vi "1dparse.vi"(5 "max0 2":u16, 7 "min0 2":u16, 10 "channel number":T1, 11 "2d intensity array output 2":i32[][](array[numeric])) -> (3 "2d intensity array output":i32[][](array[numeric]))   [LabVIEW 2016]
uses:
  controls/1d gate selection.ctl
  Drivers/Pixie4DLL.dll
panel:
  out "size(s)":i32
  out "data0":u16[](array[numeric])
  out "timeb3":u16[](array[numeric])
  out "timeb2":u16[](array[numeric])
  out "timeb1":u16[](array[numeric])
  out "timeb0":u16[](array[numeric])
  out "datab3":u16[](array[numeric])
  out "datab2":u16[](array[numeric])
  out "datab1":u16[](array[numeric])
  out "return type":u32
  out "subarray":i32[](array[numeric])
  out "size":u16
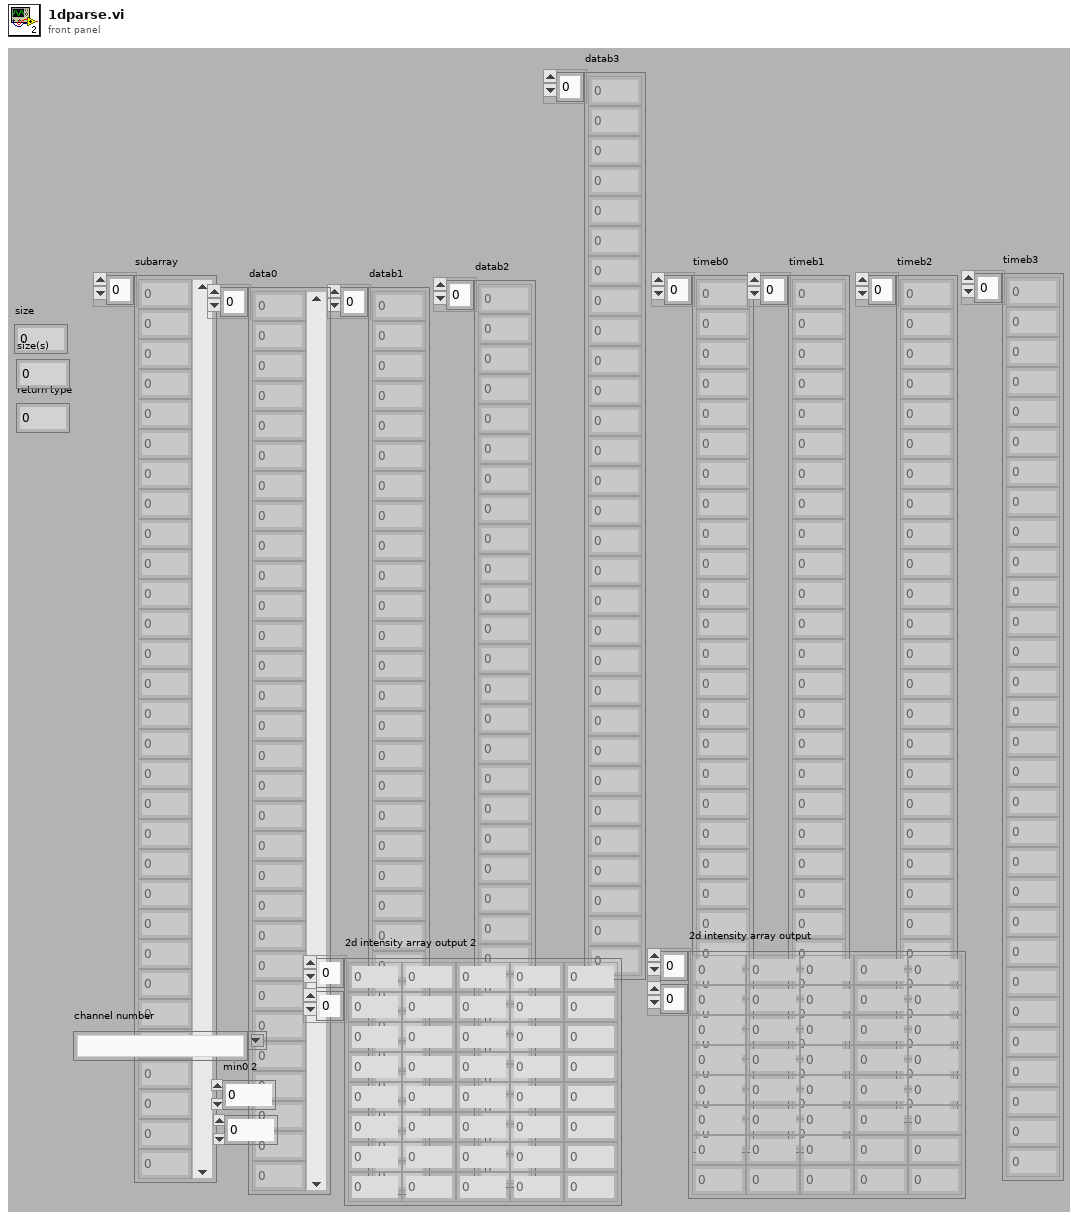
[diagram p1: front panel]
types:
  T1 = typedef "1d gate selection.ctl" = string
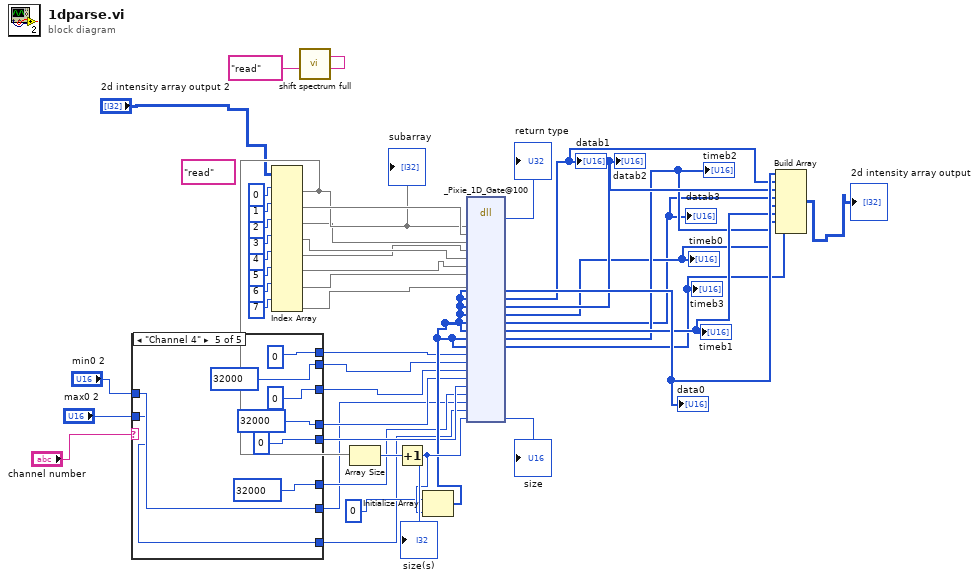
[diagram p0: block diagram]
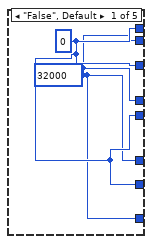
[diagram p2: hidden frame]
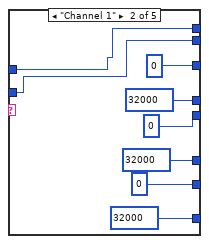
[diagram p3: hidden frame]
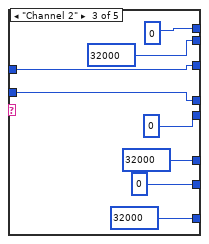
[diagram p4: hidden frame]
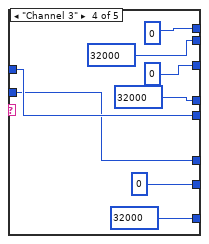
[diagram p5: hidden frame]
diagram:
  (unwired) "read" ("shift control")
  n1 = case shown="\"Channel 4\"" "channel number" {
    tunnel: [w46 w48 u16 0 ("min1") u16 0 ("min1") u16 0 ("min1")] -> w27
    tunnel: [w45 w47 u16 32000 ("min1") u16 32000 ("min1") u16 32000 ("min1")] -> w24
    tunnel: [w46 u16 0 ("min1") w56 u16 0 ("min1") u16 0 ("min1")] -> w26
    tunnel: [w45 u16 32000 ("min1") w55 u16 32000 ("min1") u16 32000 ("min1")] -> w23
    tunnel: [w46 u16 0 ("min1") u16 0 ("min1") w64 u16 0 ("min1")] -> w22
    tunnel: [w45 u16 32000 ("min1") u16 32000 ("min1") w63 u16 32000 ("min1")] -> w21
    tunnel: [w46 u16 0 ("min1") u16 0 ("min1") u16 0 ("min1") w72] -> w20
    tunnel: [w45 u16 32000 ("min1") u16 32000 ("min1") u16 32000 ("min1") w71] -> w19
    tunnel: "min0 2" -> [_ w48 w56 w64 w72]
    tunnel: "max0 2" -> [_ w47 w55 w63 w71]
    frame "False", Default {
      w45 = u16 32000 ("min1")
      w46 = u16 0 ("min1")
    }
    frame "Channel 1" {
    }
    frame "Channel 2" {
    }
    frame "Channel 3" {
    }
    frame "Channel 4" {
    }
  }
  n2 = Index Array(array="2d intensity array output 2", index (row) #1=0 ("disabled index (col)"), index (row) #2=1 ("index (col)"), index (row) #3=2 ("index (col)"), index (row) #4=3 ("index (col)"), index (row) #5=4 ("index (col)"), index (row) #6=5 ("index (col)"), index (row) #7=6 ("index (col)"), index (row) #8=7 ("index (col)")) -> (element #1=w31:i32[], element #2=w43:i32[], element #3=w8:i32[], element #4=w4:i32[], element #5=w3:i32[], element #6=w5:i32[], element #7=w42:i32[], element #8=w7:i32[])  [unwired: 8 in]
  "subarray" <- w31
  n3 = call "shift spectrum full.vi"("shift control"="read") -> ()  [unwired: 8 in, 7 out]
  n4 = Array Size(array=w31) -> (size(s)=w30:i32)
  "size(s)" <- w30
  n5 = Increment(x=w30) -> (x+1=w29:i32)
  n6 = Initialize Array(u16 0 ("min1"), w29) -> (w28:u16[])
  n7 = dll-call lib="D:/Users/wymanm/Desktop/DAQuiri - 2017a/lois/Drivers/Pixie4DLL.dll" fn="_Pixie_1D_Gate@100"("datab0"=w31, "datab1"=w43, "datab2"=w8, "datab3"=w3, "timeb0"=w4, "timeb1"=w5, "timeb2"=w42, "timeb3"=w7, "data0"=w28, "data1"=w28, "data2"=w28, "data3"=w28, "time0"=w28, "time1"=w28, "time2"=w28, "time3"=w28, "min0"=w27, "max0"=w24, "min1"=w26, "max1"=w23, "min2"=w22, "max2"=w21, "min3"=w20, "max3"=w19, "size"=w29) -> ("return type"=→"return type":u32, "data0"=w15:u16[], "data1"=w14:u16[], "data2"=w13:u16[], "data3"=w2:u16[], "time0"=w1:u16[], "time1"=w12:u16[], "time2"=w6:u16[], "time3"=w11:u16[], "size"=→"size":u16)  [unwired: 3 in, 18 out]
  "datab1" <- w14
  "datab2" <- w13
  "datab3" <- w1
  "timeb0" <- w2
  "timeb1" <- w12
  "timeb2" <- w6
  "timeb3" <- w11
  "data0" <- w15
  n8 = Build Array(w15, w14, w13, w1, w2, w12, w6, w11) -> (→"2d intensity array output":u16[][])
